vi "test Custom Report Message for Pass If Equal 1D Array (Boolean).vi"(8 "error in (no error)":errorcluster, 11 "TestCase in":refnum<class "Custom Report Message Test Case.lvclass">) -> (0 "error out":errorcluster, 3 "TestCase out":refnum<class "Custom Report Message Test Case.lvclass">)   [LabVIEW 2015, in "Custom Report Message Test Case.lvclass"]
uses:
  Custom Report Message Test Case.lvclass
  <vilib>/addons/_JKI Toolkits/VI Tester/TestCase.llb/TestCase.lvclass
  VITAC.lvlib
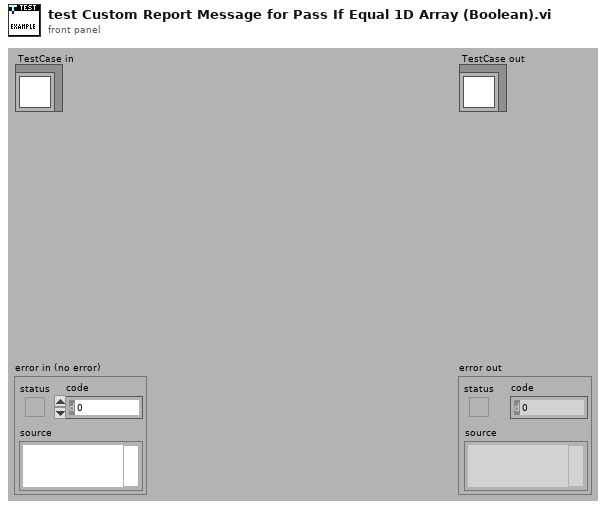
[diagram p1: front panel]
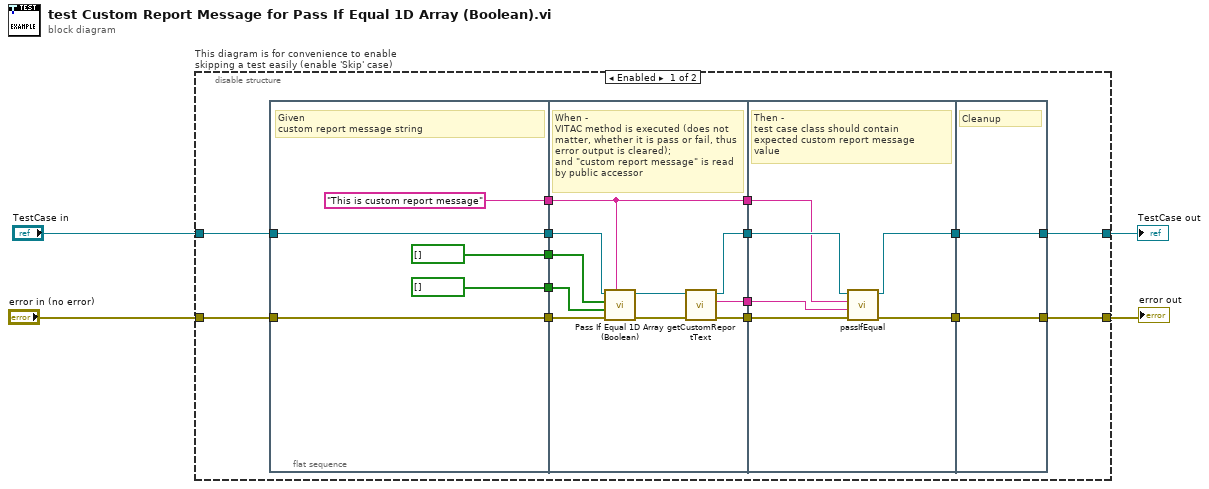
[diagram p0: block diagram]
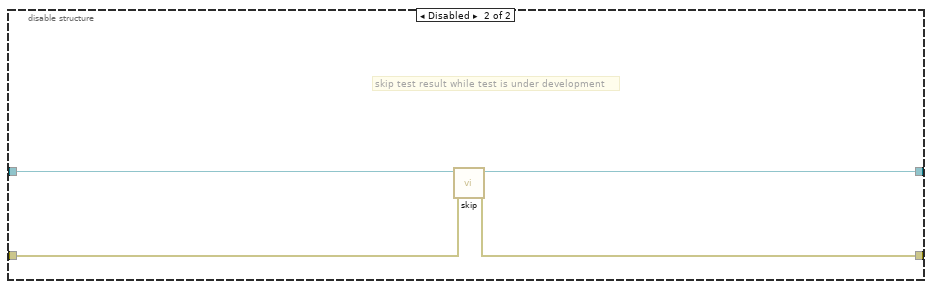
[diagram p2: hidden frame]
diagram:
  n1 = disable-structure "This diagram is for convenience to enable skipping a test easily (enable 'Skip' case)" shown="Enabled" {
    disable-tunnel: "TestCase in" -> [w11 w46]
    disable-tunnel: [w12 w44] -> w1
    disable-tunnel: [w13 w45] -> w3
    disable-tunnel: "error in (no error)" -> [w10 w43]
    frame Enabled {
      n2 = flat-sequence {
        tunnel: w10 -> [w23]
        tunnel: w11 -> [w24]
        tunnel: [w24] -> w19
        tunnel: [w23] -> w18
        tunnel: ["This is custom report message"] -> w9
        tunnel: [bool[] [] ("actual")] -> w6
        tunnel: [bool[] [] ("expected")] -> w5
        tunnel: [w32] -> w17
        tunnel: [w34] -> w16
        tunnel: w19 -> [w29]
        tunnel: w18 -> [w31]
        tunnel: w9 -> [w27]
        tunnel: [w27] -> w8
        tunnel: [w33] -> w7
        tunnel: w6 -> [w26]
        tunnel: w5 -> [w25]
        tunnel: [w39] -> w15
        tunnel: [w37] -> w14
        tunnel: w17 -> [w40]
        tunnel: w16 -> [w38]
        tunnel: w8 -> [w36]
        tunnel: w7 -> [w35]
        tunnel: [w41] -> w13
        tunnel: [w42] -> w12
        tunnel: w15 -> [w42]
        tunnel: w14 -> [w41]
        frame #0 {
          # "Given\ncustom report message string"
        }
        frame #1 {
          # "When -\nVITAC method is executed (does not matter, whether it is pass or fail, thus error output is cleared);\nand \"custom report message\" is read by public accessor"
          n3 = call "Pass If Equal 1D Array (Boolean).vi"("custom report message (\"\")"=w27, "error in (no error)"=w31, "actual"=w26, "expected"=w25, "TestCase in"=w29) -> ("error out"=w30:errorcluster, "TestCase out"=w28:refnum<class "Custom Report Message Test Case.lvclass">)  [unwired: 5 in]
          n4 = call-dynamic "getCustomReportText.vi"("error in (no error)"=w30, "TestCase in"=w28) -> ("error out"=w34:errorcluster, "customReportText"=w33:string, "TestCase out"=w32:refnum<class "Custom Report Message Test Case.lvclass">)  [unwired: 7 in]
        }
        frame #2 {
          # "Then -\ntest case class should contain \nexpected custom report message \nvalue"
          n5 = call-dynamic "passIfEqual.vi"("error in (no error)"=w38, "y"=w35, "x"=w36, "TestCase in"=w40) -> ("error out"=w37:errorcluster, "TestCase out"=w39:refnum<class "Custom Report Message Test Case.lvclass">)  [unwired: 6 in]
        }
        frame #3 {
          # "Cleanup"
        }
      }
    }
    frame Disabled {
      # "skip test result while test is under development"
      n6 = call <vilib>:"skip.vi"("error in (no error)"=w43, "TestCase in"=w46) -> ("error out"=w45:errorcluster, "TestCase out"=w44:refnum<class "Custom Report Message Test Case.lvclass">)  [unwired: 8 in]
    }
  }
  "error out" <- w3
  "TestCase out" <- w1
